vi "Name_SeqFlag.vi"() -> (1 "SeqFlag":string="StepIndex")   [LabVIEW 2016, in "SeqProcessor.lvlib"]
uses:
  SeqProcessor.lvlib
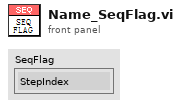
[diagram p1: front panel]
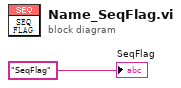
[diagram p0: block diagram]
diagram:
  "SeqFlag" <- "SeqFlag" ("Tag")
